vi "Find SVG Object.vi"(9 "Ending Delimiter":string="\"", 10 "Beginning Delimiter":string="id=\"", 11 "XML String":string) -> (1 "Ending Indices":i32[](array[numeric]), 2 "Beginning Indices":i32[](array[numeric]), 3 "Found Values":string[](array[string]))   [LabVIEW 2019, in "EditSVG.lvclass"]
uses:
  EditSVG.lvclass
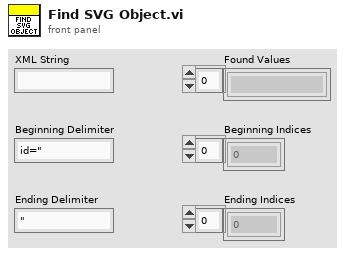
[diagram p1: front panel]
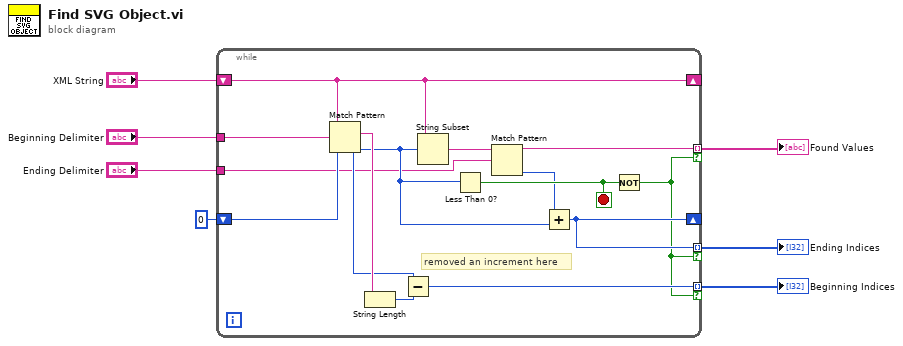
[diagram p0: block diagram]
diagram:
  n1 = while {
    shift-right: [w21] -> _
    shift-left: "XML String" -> [w21]
    shift-right: [w15] -> _
    shift-left: 0 -> [w19]
    tunnel: [w18] -> w5 mode=indexing if=w10
    tunnel: [w15] -> w3 mode=indexing if=w10
    tunnel: "Beginning Delimiter" -> [w14]
    tunnel: [w11] -> w2 mode=indexing if=w10
    tunnel: "Ending Delimiter" -> [w8]
    stop <- w17 stop-if-true
    # "removed an increment here"
    n2 = Match Pattern(string=w21, regular expression=w14, offset (0)=w19) -> (match substring=w13:string, offset past match=w12:i32)  [unwired: 2 out]
    n3 = String Length(string=w13) -> (length=w9:i32)
    n4 = Subtract(x=w12, y=w9) -> (x-y=w11:i32)
    n5 = String Subset(string=w21, offset (0)=w12) -> (substring=w20:string)  [unwired: 1 in]
    n6 = Less Than 0?(x=w12) -> (x < 0?=w17:bool)
    n7 = Match Pattern(string=w20, regular expression=w8) -> (before substring=w18:string, offset past match=w16:i32)  [unwired: 1 in, 2 out]
    n8 = Add(x=w16, y=w12) -> (x+y=w15:i32)
    n9 = Not(x=w17) -> (.not. x?=w10:bool)
  }
  "Ending Indices" <- w3
  "Beginning Indices" <- w2
  "Found Values" <- w5
